vi "Timer.vi"() -> ()   [LabVIEW 2019]
uses:
  <vilib>/ErrorRing/Error Ring.xnode
panel:
  out "Ent-ExtS":dbl[](array[numeric]) format="%#.0f"
  out "ExtS":dbl[](array[numeric]) format="%#.0f"
  out "EntS":dbl[](array[numeric]) format="%#.0f"
  out "CurrentS":dbl
  out "Cluster 2":T1
  in  "Cluster":T2
  in  "Stop":bool
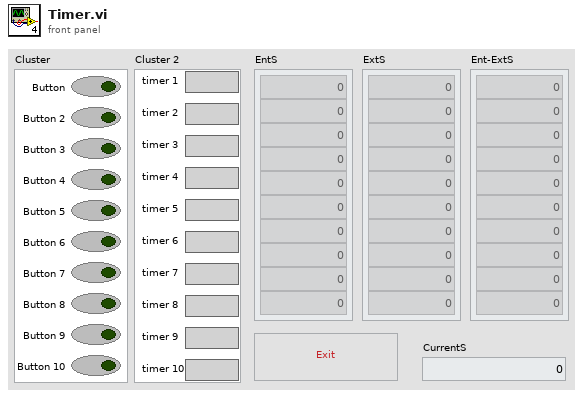
[diagram p1: front panel]
types:
  T1 = cluster{" timer 1":string, " timer 2":string, " timer 3":string, " timer 4":string, " timer 5":string, " timer 6":string, " timer 7":string, " timer 8":string, " timer 9":string, " timer 10":string}
  T2 = cluster{"Button":bool, "Button 2":bool, "Button 3":bool, "Button 4":bool, "Button 5":bool, "Button 6":bool, "Button 7":bool, "Button 8":bool, "Button 9":bool, "Button 10":bool}
  T3 = cluster{"Bay 1":bool, "Bay 2":bool, "Bay 3":bool, "Bay 4":bool, "Bay 5":bool, "Bay 6":bool, "Bay 7":bool, "Bay 8":bool, "Bay 9":bool, "Bay 10":bool}
  T4 = cluster{"[0]":string, "[1]":string, "[2]":string, "[3]":string, "[4]":string, "[5]":string, "[6]":string, "[7]":string, "[8]":string, "[9]":string}
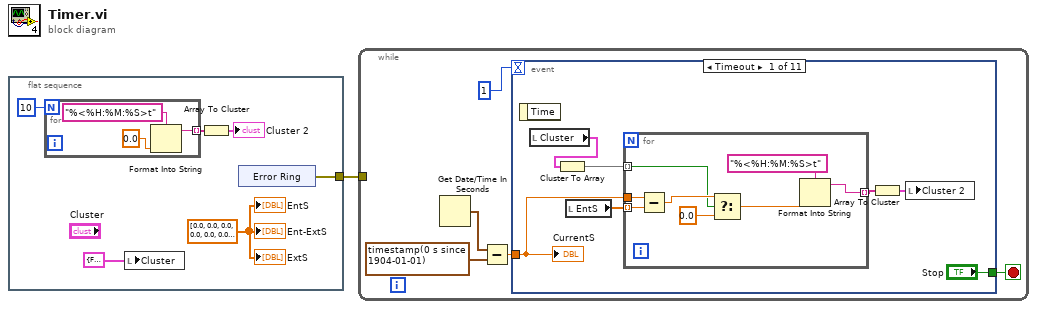
[diagram p0: block diagram]
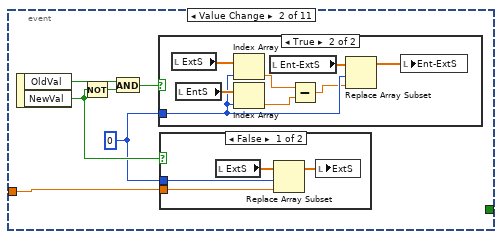
[diagram p2: hidden frame]
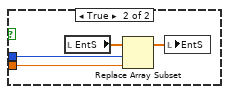
[diagram p4: hidden frame]
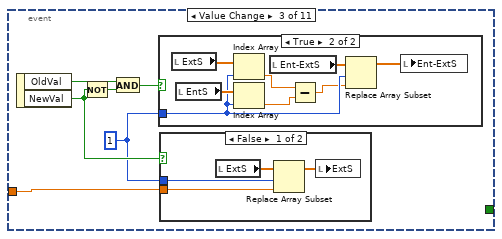
[diagram p5: hidden frame]
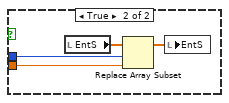
[diagram p7: hidden frame]
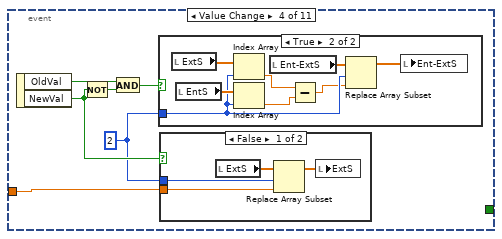
[diagram p8: hidden frame]
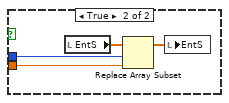
[diagram p10: hidden frame]
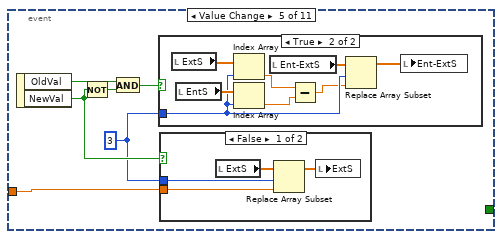
[diagram p11: hidden frame]
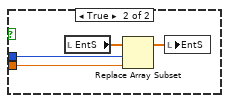
[diagram p13: hidden frame]
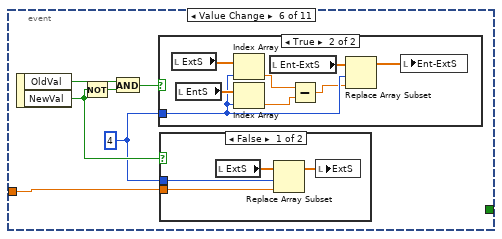
[diagram p14: hidden frame]
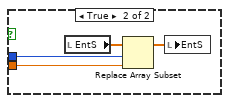
[diagram p16: hidden frame]
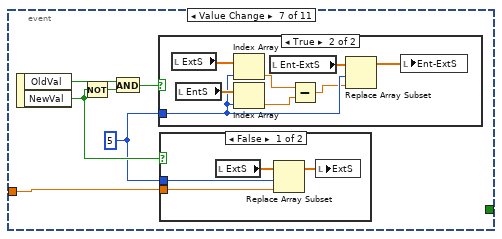
[diagram p17: hidden frame]
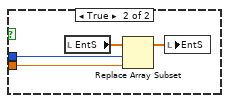
[diagram p19: hidden frame]
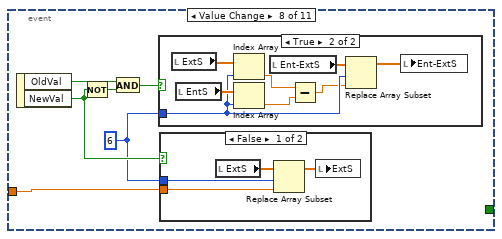
[diagram p20: hidden frame]
diagram:
  n1 = flat-sequence {
    tunnel: [w3] -> w1
    frame #0 {
      w4 = dbl[] [0.0, 0.0, 0.0, 0.0, 0.0, 0.0, 0.0, 0.0, 0.0, 0.0] ("EntS")
      n2 = for {
        N: 10 -> [_]
        tunnel: [w9] -> w6 mode=indexing
        n3 = Format Into String(format string="%<%H:%M:%S>t", 0.0 ("input 1")) -> (resulting string=w9:string)  [unwired: 2 in, 1 out]
      }
      n4 = local write "Cluster"(T3 {"Bay 1"=FALSE, "Bay 2"=FALSE, "Bay 3"=FALSE, "Bay 4"=FALSE, "Bay 5"=FALSE, "Bay 6"=FALSE, "Bay 7"=FALSE, "Bay 8"=FALSE, "Bay 9"=FALSE, "Bay 10"=FALSE} ("Occupancy")) -> ()
      n5 = Array To Cluster(array=w6) -> (cluster=→"Cluster 2":T4)
      n6 = xnode "Error Ring"() -> ("error out"=w3:errorcluster)
      "ExtS" <- w4
      "EntS" <- w4
      "Ent-ExtS" <- w4
    }
  }
  n7 = while {
    tunnel: w1 -> [_]
    stop <- w12 stop-if-true
    n8 = Get Date/Time In Seconds() -> (seconds since 1Jan1904=w15:timestamp)
    n9 = Subtract(x=w15, y=timestamp(0 s since 1904-01-01)) -> (x-y=w13:dbl)
    n10 = event shown="[0] Timeout" {
      selector: _ -> [_ _ _ _ _ _ _ _ _ _ _]
      dyn-events: _ -> [_ _ _ _ _ _ _ _ _ _ _]
      timeout: 1 -> [_ _ _ _ _ _ _ _ _ _ _]
      tunnel: w13 -> [w20 w37 w59 w81 w103 w125 w147 w169 w191 w213 w235]
      tunnel: ["Stop" _ _ _ _ _ _ _ _ _ _] -> w12
      event Timeout {
        n11 = event-data() -> ()  [unwired: 1 in, 1 out]
        n12 = local read "Cluster"() -> (w19:T2)
        n13 = Cluster To Array(cluster=w19) -> (array=w18:bool[])
        n14 = local read "EntS"() -> (w23:dbl[])
        n15 = for {
          tunnel: w23 -> [w29] mode=indexing
          tunnel: [w30] -> w22 mode=indexing
          tunnel: w20 -> [w28]
          tunnel: w18 -> [w25] mode=indexing
          n16 = Subtract(x=w28, y=w29) -> (x-y=w27:dbl)
          n17 = Select(t=w27, s=w25, f=0.0) -> (s? t:f=w24:dbl)
          n18 = Format Into String(format string="%<%H:%M:%S>t", w24) -> (resulting string=w30:string)  [unwired: 2 in, 1 out]
        }
        n19 = Array To Cluster(array=w22) -> (cluster=w21:T4)
        n20 = local write "Cluster 2"(w21) -> ()
        "CurrentS" <- w20
      }
      event "Cluster.Button": Value Change {
        w32 = 0 ("index")
        n21 = event-data() -> ("OldVal"=w36:bool, "NewVal"=w35:bool)  [unwired: 1 in]
        n22 = Not(x=w35) -> (.not. x?=w34:bool)
        n23 = And(x=w36, y=w34) -> (x .and. y?=w33:bool)
        n24 = case shown="True" w33 {
          tunnel: w32 -> [_ w42]
          frame False {
          }
          frame True {
            n25 = local read "ExtS"() -> (w45:dbl[])
            n26 = local read "EntS"() -> (w44:dbl[])
            n27 = Index Array(array=w45, index=w42) -> (element=w41:dbl)
            n28 = Index Array(array=w44, index=w42) -> (element=w40:dbl)
            n29 = local read "Ent-ExtS"() -> (w43:dbl[])
            n30 = Subtract(x=w41, y=w40) -> (x-y=w39:dbl)
            n31 = Replace Array Subset(array=w43, new element=w39, index=w42) -> (w38:dbl[])
            n32 = local write "Ent-ExtS"(w38) -> ()
          }
        }
        n33 = case shown="False" w35 {
          tunnel: w37 -> [w47 w52]
          tunnel: w32 -> [w46 w50]
          frame False {
            n34 = local read "ExtS"() -> (w49:dbl[])
            n35 = Replace Array Subset(array=w49, new element=w47, index=w46) -> (w48:dbl[])
            n36 = local write "ExtS"(w48) -> ()
          }
          frame True {
            n37 = local read "EntS"() -> (w53:dbl[])
            n38 = Replace Array Subset(array=w53, new element=w52, index=w50) -> (w51:dbl[])
            n39 = local write "EntS"(w51) -> ()
          }
        }
      }
      event "Cluster.Button 2": Value Change {
        w54 = 1 ("index")
        n40 = event-data() -> ("OldVal"=w58:bool, "NewVal"=w57:bool)  [unwired: 1 in]
        n41 = Not(x=w57) -> (.not. x?=w56:bool)
        n42 = And(x=w58, y=w56) -> (x .and. y?=w55:bool)
        n43 = case shown="True" w55 {
          tunnel: w54 -> [_ w64]
          frame False {
          }
          frame True {
            n44 = local read "ExtS"() -> (w67:dbl[])
            n45 = local read "EntS"() -> (w66:dbl[])
            n46 = Index Array(array=w67, index=w64) -> (element=w63:dbl)
            n47 = Index Array(array=w66, index=w64) -> (element=w62:dbl)
            n48 = local read "Ent-ExtS"() -> (w65:dbl[])
            n49 = Subtract(x=w63, y=w62) -> (x-y=w61:dbl)
            n50 = Replace Array Subset(array=w65, new element=w61, index=w64) -> (w60:dbl[])
            n51 = local write "Ent-ExtS"(w60) -> ()
          }
        }
        n52 = case shown="False" w57 {
          tunnel: w59 -> [w69 w74]
          tunnel: w54 -> [w68 w72]
          frame False {
            n53 = local read "ExtS"() -> (w71:dbl[])
            n54 = Replace Array Subset(array=w71, new element=w69, index=w68) -> (w70:dbl[])
            n55 = local write "ExtS"(w70) -> ()
          }
          frame True {
            n56 = local read "EntS"() -> (w75:dbl[])
            n57 = Replace Array Subset(array=w75, new element=w74, index=w72) -> (w73:dbl[])
            n58 = local write "EntS"(w73) -> ()
          }
        }
      }
      event "Cluster.Button 3": Value Change {
        w76 = 2 ("index")
        n59 = event-data() -> ("OldVal"=w80:bool, "NewVal"=w79:bool)  [unwired: 1 in]
        n60 = Not(x=w79) -> (.not. x?=w78:bool)
        n61 = And(x=w80, y=w78) -> (x .and. y?=w77:bool)
        n62 = case shown="True" w77 {
          tunnel: w76 -> [_ w86]
          frame False {
          }
          frame True {
            n63 = local read "ExtS"() -> (w89:dbl[])
            n64 = local read "EntS"() -> (w88:dbl[])
            n65 = Index Array(array=w89, index=w86) -> (element=w85:dbl)
            n66 = Index Array(array=w88, index=w86) -> (element=w84:dbl)
            n67 = local read "Ent-ExtS"() -> (w87:dbl[])
            n68 = Subtract(x=w85, y=w84) -> (x-y=w83:dbl)
            n69 = Replace Array Subset(array=w87, new element=w83, index=w86) -> (w82:dbl[])
            n70 = local write "Ent-ExtS"(w82) -> ()
          }
        }
        n71 = case shown="False" w79 {
          tunnel: w81 -> [w91 w96]
          tunnel: w76 -> [w90 w94]
          frame False {
            n72 = local read "ExtS"() -> (w93:dbl[])
            n73 = Replace Array Subset(array=w93, new element=w91, index=w90) -> (w92:dbl[])
            n74 = local write "ExtS"(w92) -> ()
          }
          frame True {
            n75 = local read "EntS"() -> (w97:dbl[])
            n76 = Replace Array Subset(array=w97, new element=w96, index=w94) -> (w95:dbl[])
            n77 = local write "EntS"(w95) -> ()
          }
        }
      }
      event "Cluster.Button 4": Value Change {
        w98 = 3 ("index")
        n78 = event-data() -> ("OldVal"=w102:bool, "NewVal"=w101:bool)  [unwired: 1 in]
        n79 = Not(x=w101) -> (.not. x?=w100:bool)
        n80 = And(x=w102, y=w100) -> (x .and. y?=w99:bool)
        n81 = case shown="True" w99 {
          tunnel: w98 -> [_ w108]
          frame False {
          }
          frame True {
            n82 = local read "ExtS"() -> (w111:dbl[])
            n83 = local read "EntS"() -> (w110:dbl[])
            n84 = Index Array(array=w111, index=w108) -> (element=w107:dbl)
            n85 = Index Array(array=w110, index=w108) -> (element=w106:dbl)
            n86 = local read "Ent-ExtS"() -> (w109:dbl[])
            n87 = Subtract(x=w107, y=w106) -> (x-y=w105:dbl)
            n88 = Replace Array Subset(array=w109, new element=w105, index=w108) -> (w104:dbl[])
            n89 = local write "Ent-ExtS"(w104) -> ()
          }
        }
        n90 = case shown="False" w101 {
          tunnel: w103 -> [w113 w118]
          tunnel: w98 -> [w112 w116]
          frame False {
            n91 = local read "ExtS"() -> (w115:dbl[])
            n92 = Replace Array Subset(array=w115, new element=w113, index=w112) -> (w114:dbl[])
            n93 = local write "ExtS"(w114) -> ()
          }
          frame True {
            n94 = local read "EntS"() -> (w119:dbl[])
            n95 = Replace Array Subset(array=w119, new element=w118, index=w116) -> (w117:dbl[])
            n96 = local write "EntS"(w117) -> ()
          }
        }
      }
      event "Cluster.Button 5": Value Change {
        w120 = 4 ("index")
        n97 = event-data() -> ("OldVal"=w124:bool, "NewVal"=w123:bool)  [unwired: 1 in]
        n98 = Not(x=w123) -> (.not. x?=w122:bool)
        n99 = And(x=w124, y=w122) -> (x .and. y?=w121:bool)
        n100 = case shown="True" w121 {
          tunnel: w120 -> [_ w130]
          frame False {
          }
          frame True {
            n101 = local read "ExtS"() -> (w133:dbl[])
            n102 = local read "EntS"() -> (w132:dbl[])
            n103 = Index Array(array=w133, index=w130) -> (element=w129:dbl)
            n104 = Index Array(array=w132, index=w130) -> (element=w128:dbl)
            n105 = local read "Ent-ExtS"() -> (w131:dbl[])
            n106 = Subtract(x=w129, y=w128) -> (x-y=w127:dbl)
            n107 = Replace Array Subset(array=w131, new element=w127, index=w130) -> (w126:dbl[])
            n108 = local write "Ent-ExtS"(w126) -> ()
          }
        }
        n109 = case shown="False" w123 {
          tunnel: w125 -> [w135 w140]
          tunnel: w120 -> [w134 w138]
          frame False {
            n110 = local read "ExtS"() -> (w137:dbl[])
            n111 = Replace Array Subset(array=w137, new element=w135, index=w134) -> (w136:dbl[])
            n112 = local write "ExtS"(w136) -> ()
          }
          frame True {
            n113 = local read "EntS"() -> (w141:dbl[])
            n114 = Replace Array Subset(array=w141, new element=w140, index=w138) -> (w139:dbl[])
            n115 = local write "EntS"(w139) -> ()
          }
        }
      }
      event "Cluster.Button 6": Value Change {
        w142 = 5 ("index")
        n116 = event-data() -> ("OldVal"=w146:bool, "NewVal"=w145:bool)  [unwired: 1 in]
        n117 = Not(x=w145) -> (.not. x?=w144:bool)
        n118 = And(x=w146, y=w144) -> (x .and. y?=w143:bool)
        n119 = case shown="True" w143 {
          tunnel: w142 -> [_ w152]
          frame False {
          }
          frame True {
            n120 = local read "ExtS"() -> (w155:dbl[])
            n121 = local read "EntS"() -> (w154:dbl[])
            n122 = Index Array(array=w155, index=w152) -> (element=w151:dbl)
            n123 = Index Array(array=w154, index=w152) -> (element=w150:dbl)
            n124 = local read "Ent-ExtS"() -> (w153:dbl[])
            n125 = Subtract(x=w151, y=w150) -> (x-y=w149:dbl)
            n126 = Replace Array Subset(array=w153, new element=w149, index=w152) -> (w148:dbl[])
            n127 = local write "Ent-ExtS"(w148) -> ()
          }
        }
        n128 = case shown="False" w145 {
          tunnel: w147 -> [w157 w162]
          tunnel: w142 -> [w156 w160]
          frame False {
            n129 = local read "ExtS"() -> (w159:dbl[])
            n130 = Replace Array Subset(array=w159, new element=w157, index=w156) -> (w158:dbl[])
            n131 = local write "ExtS"(w158) -> ()
          }
          frame True {
            n132 = local read "EntS"() -> (w163:dbl[])
            n133 = Replace Array Subset(array=w163, new element=w162, index=w160) -> (w161:dbl[])
            n134 = local write "EntS"(w161) -> ()
          }
        }
      }
      event "Cluster.Button 7": Value Change {
        w164 = 6 ("index")
        n135 = event-data() -> ("OldVal"=w168:bool, "NewVal"=w167:bool)  [unwired: 1 in]
        n136 = Not(x=w167) -> (.not. x?=w166:bool)
        n137 = And(x=w168, y=w166) -> (x .and. y?=w165:bool)
        n138 = case shown="True" w165 {
          tunnel: w164 -> [_ w174]
          frame False {
          }
          frame True {
            n139 = local read "ExtS"() -> (w177:dbl[])
            n140 = local read "EntS"() -> (w176:dbl[])
            n141 = Index Array(array=w177, index=w174) -> (element=w173:dbl)
            n142 = Index Array(array=w176, index=w174) -> (element=w172:dbl)
            n143 = local read "Ent-ExtS"() -> (w175:dbl[])
            n144 = Subtract(x=w173, y=w172) -> (x-y=w171:dbl)
            n145 = Replace Array Subset(array=w175, new element=w171, index=w174) -> (w170:dbl[])
            n146 = local write "Ent-ExtS"(w170) -> ()
          }
        }
        n147 = case shown="False" w167 {
          tunnel: w169 -> [w179 w184]
          tunnel: w164 -> [w178 w182]
          frame False {
            n148 = local read "ExtS"() -> (w181:dbl[])
            n149 = Replace Array Subset(array=w181, new element=w179, index=w178) -> (w180:dbl[])
            n150 = local write "ExtS"(w180) -> ()
          }
          frame True {
            n151 = local read "EntS"() -> (w185:dbl[])
            n152 = Replace Array Subset(array=w185, new element=w184, index=w182) -> (w183:dbl[])
            n153 = local write "EntS"(w183) -> ()
          }
        }
      }
      event "Cluster.Button 8": Value Change {
        w186 = 7 ("index")
        n154 = event-data() -> ("OldVal"=w190:bool, "NewVal"=w189:bool)  [unwired: 1 in]
        n155 = Not(x=w189) -> (.not. x?=w188:bool)
        n156 = And(x=w190, y=w188) -> (x .and. y?=w187:bool)
        n157 = case shown="True" w187 {
          tunnel: w186 -> [_ w196]
          frame False {
          }
          frame True {
            n158 = local read "ExtS"() -> (w199:dbl[])
            n159 = local read "EntS"() -> (w198:dbl[])
            n160 = Index Array(array=w199, index=w196) -> (element=w195:dbl)
            n161 = Index Array(array=w198, index=w196) -> (element=w194:dbl)
            n162 = local read "Ent-ExtS"() -> (w197:dbl[])
            n163 = Subtract(x=w195, y=w194) -> (x-y=w193:dbl)
            n164 = Replace Array Subset(array=w197, new element=w193, index=w196) -> (w192:dbl[])
            n165 = local write "Ent-ExtS"(w192) -> ()
          }
        }
        n166 = case shown="False" w189 {
          tunnel: w191 -> [w201 w206]
          tunnel: w186 -> [w200 w204]
          frame False {
            n167 = local read "ExtS"() -> (w203:dbl[])
            n168 = Replace Array Subset(array=w203, new element=w201, index=w200) -> (w202:dbl[])
            n169 = local write "ExtS"(w202) -> ()
          }
          frame True {
            n170 = local read "EntS"() -> (w207:dbl[])
            n171 = Replace Array Subset(array=w207, new element=w206, index=w204) -> (w205:dbl[])
            n172 = local write "EntS"(w205) -> ()
          }
        }
      }
      event "Cluster.Button 9": Value Change {
        w208 = 8 ("index")
        n173 = event-data() -> ("OldVal"=w212:bool, "NewVal"=w211:bool)  [unwired: 1 in]
        n174 = Not(x=w211) -> (.not. x?=w210:bool)
        n175 = And(x=w212, y=w210) -> (x .and. y?=w209:bool)
        n176 = case shown="True" w209 {
          tunnel: w208 -> [_ w218]
          frame False {
          }
          frame True {
            n177 = local read "ExtS"() -> (w221:dbl[])
            n178 = local read "EntS"() -> (w220:dbl[])
            n179 = Index Array(array=w221, index=w218) -> (element=w217:dbl)
            n180 = Index Array(array=w220, index=w218) -> (element=w216:dbl)
            n181 = local read "Ent-ExtS"() -> (w219:dbl[])
            n182 = Subtract(x=w217, y=w216) -> (x-y=w215:dbl)
            n183 = Replace Array Subset(array=w219, new element=w215, index=w218) -> (w214:dbl[])
            n184 = local write "Ent-ExtS"(w214) -> ()
          }
        }
        n185 = case shown="False" w211 {
          tunnel: w213 -> [w223 w228]
          tunnel: w208 -> [w222 w226]
          frame False {
            n186 = local read "ExtS"() -> (w225:dbl[])
            n187 = Replace Array Subset(array=w225, new element=w223, index=w222) -> (w224:dbl[])
            n188 = local write "ExtS"(w224) -> ()
          }
          frame True {
            n189 = local read "EntS"() -> (w229:dbl[])
            n190 = Replace Array Subset(array=w229, new element=w228, index=w226) -> (w227:dbl[])
            n191 = local write "EntS"(w227) -> ()
          }
        }
      }
      event "Cluster.Button 10": Value Change {
        w230 = 9 ("index")
        n192 = event-data() -> ("OldVal"=w234:bool, "NewVal"=w233:bool)  [unwired: 1 in]
        n193 = Not(x=w233) -> (.not. x?=w232:bool)
        n194 = And(x=w234, y=w232) -> (x .and. y?=w231:bool)
        n195 = case shown="True" w231 {
          tunnel: w230 -> [_ w240]
          frame False {
          }
          frame True {
            n196 = local read "ExtS"() -> (w243:dbl[])
            n197 = local read "EntS"() -> (w242:dbl[])
            n198 = Index Array(array=w243, index=w240) -> (element=w239:dbl)
            n199 = Index Array(array=w242, index=w240) -> (element=w238:dbl)
            n200 = local read "Ent-ExtS"() -> (w241:dbl[])
            n201 = Subtract(x=w239, y=w238) -> (x-y=w237:dbl)
            n202 = Replace Array Subset(array=w241, new element=w237, index=w240) -> (w236:dbl[])
            n203 = local write "Ent-ExtS"(w236) -> ()
          }
        }
        n204 = case shown="False" w233 {
          tunnel: w235 -> [w245 w250]
          tunnel: w230 -> [w244 w248]
          frame False {
            n205 = local read "ExtS"() -> (w247:dbl[])
            n206 = Replace Array Subset(array=w247, new element=w245, index=w244) -> (w246:dbl[])
            n207 = local write "ExtS"(w246) -> ()
          }
          frame True {
            n208 = local read "EntS"() -> (w251:dbl[])
            n209 = Replace Array Subset(array=w251, new element=w250, index=w248) -> (w249:dbl[])
            n210 = local write "EntS"(w249) -> ()
          }
        }
      }
    }
  }
